vi "Steering Motor Encoder Read.vi"(9 "Flag Steering Encoder":dbl, 10 "Reset Counter":bool, 11 "Error In":errorcluster) -> (1 "Encoder output":T1, 3 "Error Out":errorcluster)   [LabVIEW 2021]
uses:
  <vilib>/myRIO/Common/Instrument Driver Framework/myRIO v1.0/Encoder/typedefs/Encoder Signal Mode.ctl
  <vilib>/myRIO/Instrument Drivers/Onboard IO/Encoder/typedefs/Encoder Reference.ctl
  <vilib>/myRIO/Common/Instrument Driver Framework/Utilities/typedefs/myRIO Generic Hardware Reference.ctl
  <vilib>/myRIO/Common/Instrument Driver Framework/Utilities/typedefs/Hardware Version Enum.ctl
  <vilib>/myRIO/Common/Instrument Driver Framework/Utilities/typedefs/myRIO v1.0 Reference.ctl
  <vilib>/myRIO/Common/Instrument Driver Framework/Utilities/typedefs/Generic FPGA Reference.ctl
  <vilib>/myRIO/Common/Instrument Driver Framework/myRIO v1.0/Encoder/typedefs/Encoder Channels Enum.ctl
  <vilib>/myRIO/Common/Instrument Driver Framework/myRIO v1.0/Encoder/typedefs/Encoder Configuration v1.0.ctl
  <vilib>/userdefined/High Color/nirio_resource_hc.ctl
  <vilib>/myRIO/Common/Instrument Driver Framework/Utilities/vis/Is FPGA Ref Available.vi
  <vilib>/myRIO/Common/Instrument Driver Framework/myRIO v1.0/Encoder/vis/myRIO v1.1 Open Encoder.vi
  <vilib>/myRIO/Instrument Drivers/Onboard IO/Encoder/vis/Read.vi
  <vilib>/myRIO/Common/Instrument Driver Framework/Utilities/vis/Validate Channels.vi
  <vilib>/myRIO/Common/Instrument Driver Framework/myRIO v1.0/Encoder/vis/myRIO v1.0 Reserve Encoder.vi
  <vilib>/myRIO/Common/Instrument Driver Framework/myRIO v1.0/Encoder/vis/myRIO v1.0 Build MUX Configuration Encoder.vi
  <vilib>/myRIO/Common/Instrument Driver Framework/myRIO v1.0/Resource Manager/vis/myRIO v1.0 Reserve Channel List.vi
  <vilib>/myRIO/Common/Instrument Driver Framework/myRIO v1.0/Resource Manager/vis/myRIO v1.0 Create Configuration List.vi
  <vilib>/myRIO/Common/Instrument Driver Framework/myRIO v1.0/Resource Manager/vis/myRIO v1.0 Reserve Channel.vi
  <vilib>/myRIO/Common/Instrument Driver Framework/myRIO v1.0/Resource Manager/vis/myRIO v1.0 Unreserve Channel.vi
  <vilib>/myRIO/Common/Instrument Driver Framework/myRIO v1.0/Resource Manager/vis/myRIO v1.0 Build Mutex Name.vi
  <vilib>/Utility/VariantDataType/GetNumericInfo.vi
  <vilib>/Utility/error.llb/Error Cluster From Error Code.vi
  <vilib>/myRIO/Common/Instrument Driver Framework/myRIO v1.0/myRIO v1.1 Open.vi
  <vilib>/myRIO/Common/Instrument Driver Framework/Utilities/vis/IO Manager.vi
  <vilib>/myRIO/Common/Instrument Driver Framework/Utilities/vis/Configuration Manager.vi
  <vilib>/myRIO/Common/Instrument Driver Framework/myRIO v1.0/Resource Manager/vis/myRIO v1.0 Configure IO.vi
  <vilib>/myRIO/Common/Instrument Driver Framework/myRIO v1.0/myRIO v1.0 Close.vi
  <vilib>/myRIO/Common/Instrument Driver Framework/myRIO v1.0/Encoder/vis/myRIO v1.0 Configure Encoder.vi
  <vilib>/myRIO/Common/Instrument Driver Framework/myRIO v1.0/Encoder/vis/myRIO v1.0 Read Encoder.vi
  <vilib>/myRIO/Express VI/Onboard IO/Encoder/Encoder Express VI.xnode
  <vilib>/myRIO/Instrument Drivers/Onboard IO/Encoder/vis/myRIO Encoder Open.xnode
  <vilib>/myRIO/Common/Instrument Driver Framework/myRIO v1.0/Encoder/typedefs/Encoder Count Direction Enum.ctl
  <vilib>/myRIO/Instrument Drivers/Onboard IO/Encoder/Encoder.lvlib
panel:
  out "Encoder position (deg)":dbl
  out "Cluster":T2={"Steering Pully Gear Ratio"=1.0, "Steering Motor Gear Ratio"=1.0, "Steering Encoder CPR"=1024.0}
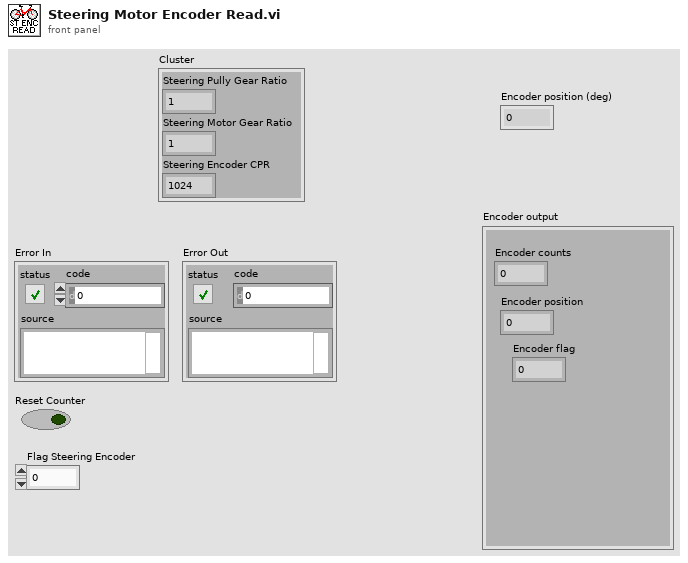
[diagram p1: front panel]
types:
  T1 = cluster{"Encoder counts":dbl, "Encoder position":dbl, "Encoder flag":dbl}
  T2 = cluster{"Steering Pully Gear Ratio":dbl, "Steering Motor Gear Ratio":dbl, "Steering Encoder CPR":dbl}
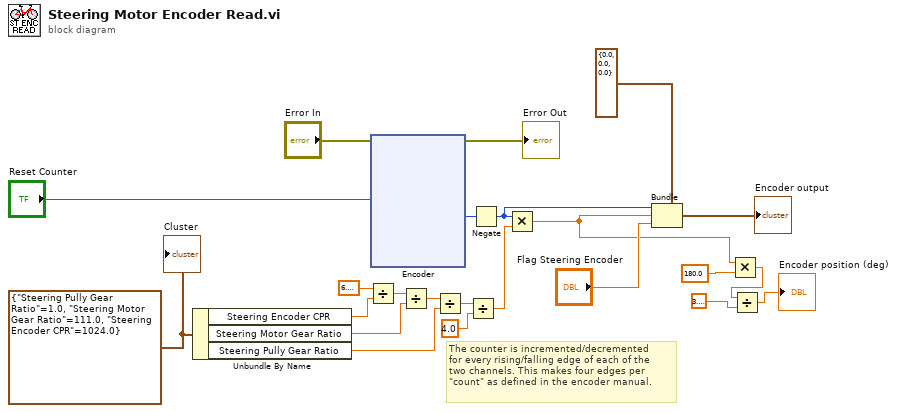
[diagram p0: block diagram]
diagram:
  w8 = T2 {"Steering Pully Gear Ratio"=1.0, "Steering Motor Gear Ratio"=111.0, "Steering Encoder CPR"=1024.0}
  # "The counter is incremented/decremented\nfor every rising/falling edge of each of the\ntwo channels. This makes four edges per\n\"count\" as defined in the encoder manual."
  n1 = Unbundle By Name(w8) -> ("Steering Encoder CPR"=w19:dbl, "Steering Motor Gear Ratio"=w17:dbl, "Steering Pully Gear Ratio"=w15:dbl)
  n2 = Divide(x=6.283185307179586, y=w19) -> (x/y=w18:dbl)
  n3 = xnode "Encoder"("Reset Counter"="Reset Counter", "error in (no error)"="Error In") -> ("Counter Value"=w22:i32, "error out"=→"Error Out":errorcluster)  [unwired: 2 out]
  n4 = Divide(x=w18, y=w17) -> (x/y=w16:dbl)
  n5 = Divide(x=w16, y=w15) -> (x/y=w14:dbl)
  n6 = Divide(x=w14, y=4.0) -> (x/y=w13:dbl)
  n7 = Negate(x=w22) -> (-x=w21:i32)
  n8 = Multiply(x=w21, y=w13) -> (x*y=w3:dbl)
  n9 = Bundle(cluster=cluster{dbl, dbl, dbl} {0.0, 0.0, 0.0}, w21, w3, "Flag Steering Encoder") -> (→"Encoder output":cluster{dbl, dbl, dbl})
  n10 = Multiply(x=w3, y=180.0) -> (x*y=w5:dbl)
  n11 = Divide(x=w5, y=3.141592653589793) -> (x/y=→"Encoder position (deg)":dbl)
  "Cluster" <- w8
